vi "Mode_Button_State.vi"(8 "error in (no error)":errorcluster) -> (0 "error out":errorcluster, 3 "Boolean":bool)   [LabVIEW 2014]
uses:
  <userlib>/UCSD Robotics Lab/Robotics-Cape/LV/libroboticscape.lvlib
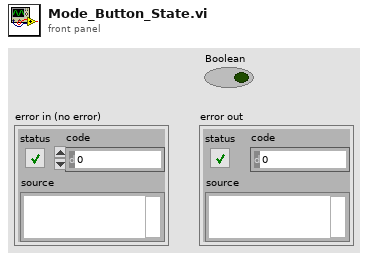
[diagram p1: front panel]
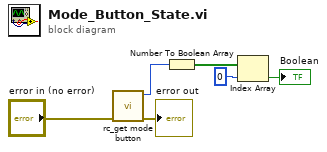
[diagram p0: block diagram]
diagram:
  n1 = call <userlib>:"rc_get mode button.vi"("error in (no error)"="error in (no error)") -> ("error out"=→"error out":errorcluster, "function return"=w3:u32)  [unwired: 9 in]
  n2 = Number To Boolean Array(number=w3) -> (Boolean array=w4:bool[])
  n3 = Index Array(array=w4, index=0) -> (element=→"Boolean":bool)
